vi "Read HV On Relay.vi"(4 "error in":errorcluster) -> (0 "error out":errorcluster, 2 "HV On Relay":bool)   [LabVIEW 2015]
uses:
  <vilib>/DAQmx/read.llb/DAQmx Read (Digital Bool 1Line 1Point).vi
  <vilib>/DAQmx/write.llb/DAQmx Write (Digital Bool 1Line 1Point).vi
  <vilib>/DAQmx/miscellaneous.llb/DAQmx Fill In Error Info.vi
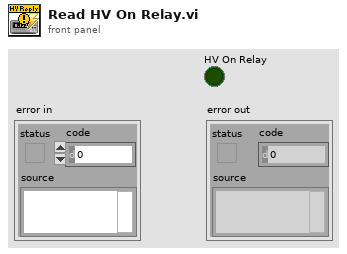
[diagram p1: front panel]
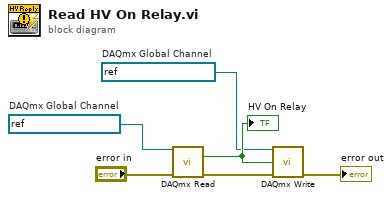
[diagram p0: block diagram]
diagram:
  w3 = refnum<k21> "DO8 HV ON LED"  # DAQmx Global Channel
  w4 = refnum<k21> "DI7 HV On reply"  # DAQmx Global Channel
  n1 = call-poly <vilib>:"DAQmx Read.vi"("task/channels in"=w4, "error in"="error in") -> ("data"=w5:bool, "error out"=w6:errorcluster)  [unwired: 11 in, 1 out]
  "HV On Relay" <- w5
  n2 = call-poly <vilib>:"DAQmx Write.vi"("task/channels in"=w3, "data"=w5, "error in"=w6) -> ("error out"=→"error out":errorcluster)  [unwired: 10 in, 2 out]
